vi "Test30ISOmoins.vi"(8 "errin":errorcluster, 9 "L2T":T1, 10 "Value":string, 11 "SN":string) -> (0 "error out":errorcluster, 3 "ISO-":string)   [LabVIEW 2020]
uses:
  <vilib>/regexp/Match Regular Expression.xnode
  Ctrl/L2T.ctl
panel:
  # "Pre DCIR_____________________________________"
  # "intra DCIR_____________________________________"
  # "Post DCIR_____________________________________"
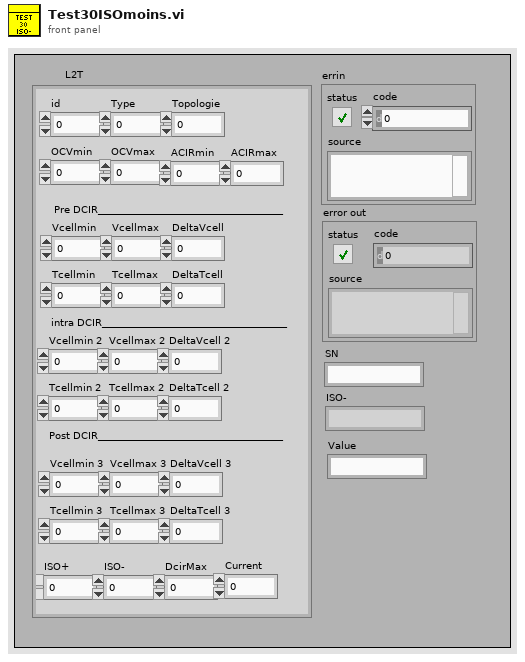
[diagram p1: front panel]
types:
  T1 = typedef "L2T.ctl" = cluster{"id":dbl, "Type":dbl, "OCVmin":dbl, "OCVmax":dbl, "ACIRmin":dbl, "ACIRmax":dbl, "Vcellmin":dbl, "Vcellmax":dbl, "DeltaVcell":dbl, "Tcellmin":dbl, "Tcellmax":dbl, "DeltaTcell":dbl, "ISO+":dbl, "ISO-":dbl, "DcirMax":dbl, "Current":dbl, "Topologie":dbl, "Vcellmin 2":dbl, "Vcellmax 2":dbl, "DeltaVcell 2":dbl, "Tcellmin 2":dbl, "Tcellmax 2":dbl, "DeltaTcell 2":dbl, "Vcellmin 3":dbl, "Vcellmax 3":dbl, "DeltaVcell 3":dbl, "Tcellmin 3":dbl, "Tcellmax 3":dbl, "DeltaTcell 3":dbl}
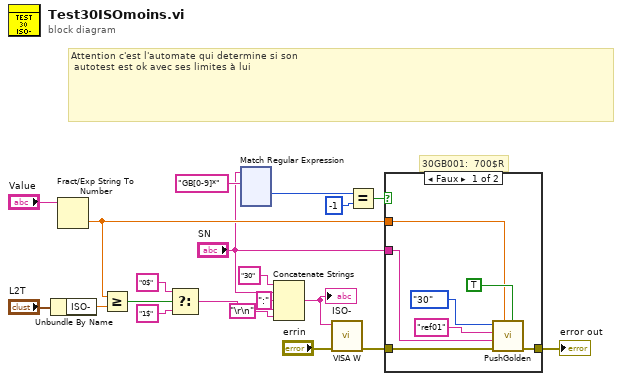
[diagram p0: block diagram]
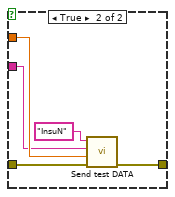
[diagram p2: hidden frame]
diagram:
  # "Attention c'est l'automate qui determine si son\n autotest est ok avec ses limites à lui"
  # "30GB001:  700$R"
  n1 = Unbundle By Name("L2T") -> ("ISO-"=w17:dbl)
  n2 = Fract/Exp String To Number(string="Value") -> (number=w18:dbl)  [unwired: 3 in, 1 out]
  n3 = Greater Or Equal?(x=w18, y=w17) -> (x >= y?=w7:bool)
  n4 = Select(t="0$" ("chaîne"), s=w7, f="1$" ("chaîne")) -> (s? t:f=w9:string)
  n5 = xnode "Match Regular Expression"("input string"="SN", "regular expression"="GB[0-9]*") -> ("offset past match"=w14:i32)  [unwired: 4 in, 4 out]
  n6 = Concatenate Strings("30" ("chaîne"), "SN", ":" ("string"), w9, "\r\n") -> (w10:string)
  "ISO-" <- w10
  n7 = call "VISA W.vi"("errin"="errin", "Chaîne"=w10) -> ("errout"=w2:errorcluster)  [unwired: 9 in]
  n8 = Equal?(x=w14, y=-1) -> (x = y?=w11:bool)
  n9 = case shown="Faux" w11 {
    tunnel: w2 -> [w24 w28]
    tunnel: [w23 w32] -> w20
    tunnel: w18 -> [w22 w31]
    tunnel: "SN" -> [w21 w29]
    frame False {
      n10 = call "PushGolden.vi"("isInt?"=TRUE, "Value"=w22, "errin"=w24, "SN"=w21, "refFile"="ref01", "testnumber"=enum16{"50", "40", "30", "20", "11", "10", ""}."30") -> ("error out"=w23:errorcluster)  [unwired: 5 in]
    }
    frame True {
      n11 = call "Send test DATA.vi"("errin"=w28, "Value"=w31, "SN"=w29, "test"="InsuN") -> ("error out"=w32:errorcluster)  [unwired: 7 in]
    }
  }
  "error out" <- w20
